vi "SubVI_ALD-Process-Step_Pulse_V16.vi"(0 "error in (no error)":errorcluster, 1 "Mod8 DAQ Name":tag, 2 "Mod7 DAQ Name":tag, 3 "Precursor Dose Array":T2={"Mod7"=[FALSE, FALSE, FALSE, FALSE, FALSE, FALSE, FALSE, FALSE], "Mod8"=[FALSE, FALSE, FALSE, FALSE, FALSE, FALSE, FALSE, FALSE]}, 5 "Precursor-i":i32, 7 "Precursor-i name":string, 9 "Dose Time (sec)":dbl, 12 "ProcessStep Input Cluster":T1, 14 "Recipe Step \nNumber":i32) -> (4 "error out":errorcluster, 8 "Dose Start Timestamp":timestamp, 15 "Execution Aborted \nDuring This Recipe Step?":bool)   [LabVIEW 2026]
uses:
  CTRL_DO Boolean Array Cluster_V16.ctl
panel:
  out "Dose Start Time":dbl
  # "NEED TO UPDATE SUBVI DESCRIPTION"
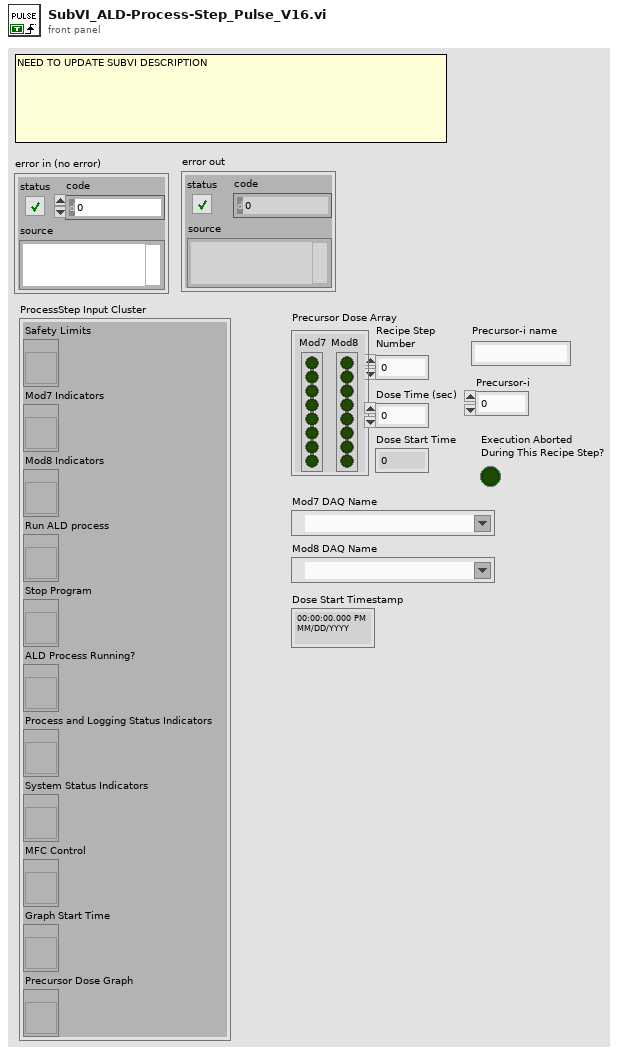
[diagram p1: front panel]
types:
  T1 = cluster{"Safety Limits":refnum<vi>, "Mod7 Indicators ":refnum<vi>, "Mod8 Indicators":refnum<vi>, "Run ALD process":refnum<vi>, "Stop Program":refnum<vi>, "ALD Process Running?":refnum<vi>, "Process and Logging Status Indicators":refnum<vi>, "System Status Indicators":refnum<vi>, "MFC Control":refnum<vi>, "Graph Start Time":refnum<vi>, "Precursor Dose Graph":refnum<vi>}
  T2 = typedef "CTRL_DO Boolean Array Cluster_V16.ctl" = cluster{"Mod7":bool[], "Mod8":bool[]}
  T3 = typedef "CTRL_ProcessLoggingStatusIndicator_V14.ctl" = cluster{"ALD Process Status:":string, "Logging Data to:":path, "Process Start Time:":string, "Process End Time:":string, "Steps Completed:":string}
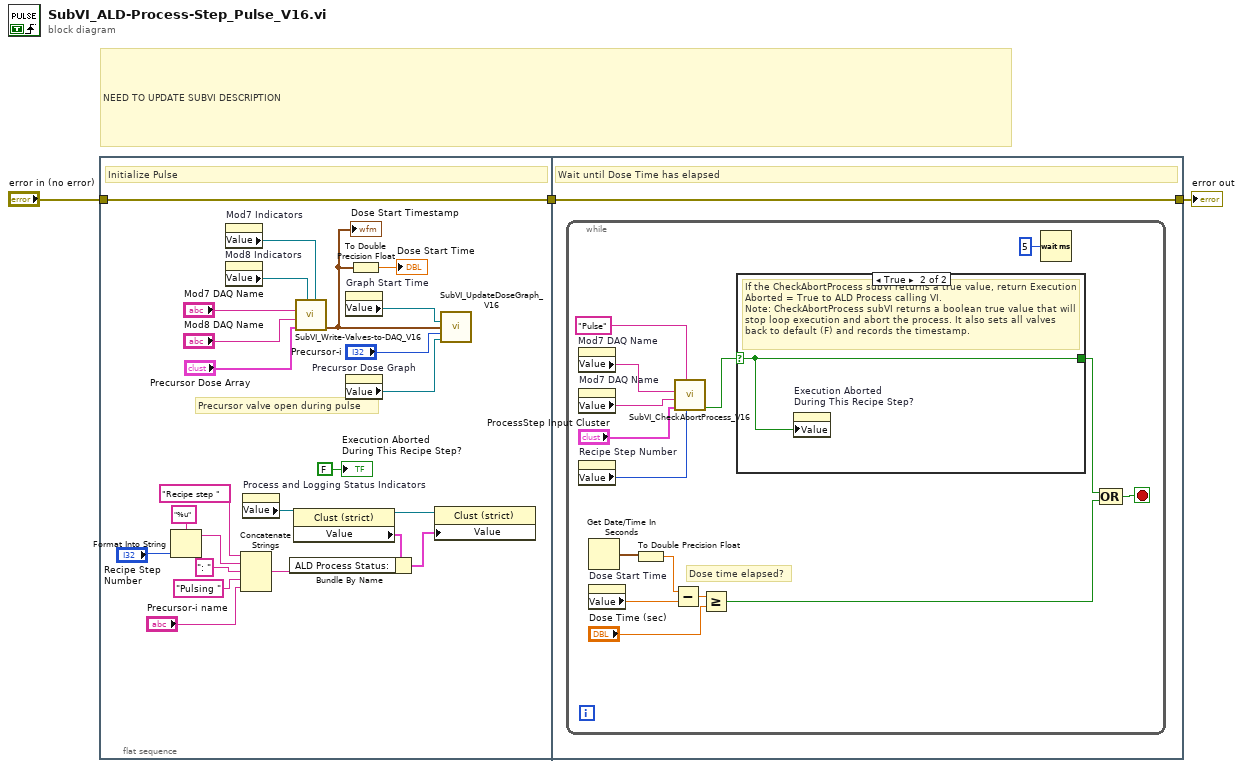
[diagram p0: block diagram]
diagram:
  # "NEED TO UPDATE SUBVI DESCRIPTION"
  n1 = flat-sequence {
    tunnel: "error in (no error)" -> [w26]
    tunnel: [w26] -> w1
    tunnel: [w28] -> w2
    tunnel: w1 -> [w28]
    frame #0 {
      # "Precursor valve open during pulse"
      # "Initialize Pulse"
      n2 = Format Into String(format string="%u", "Recipe Step \nNumber") -> (resulting string=w21:string)  [unwired: 2 in, 1 out]
      n3 = property on="Mod7 Indicators" class="LVObjRef (strict)"() -> ("Value"=w10:refnum<vi>)  [unwired: 2 in, 2 out]
      n4 = property on="Mod8 Indicators" class="LVObjRef (strict)"() -> ("Value"=w11:refnum<vi>)  [unwired: 2 in, 2 out]
      n5 = Concatenate Strings("Recipe step ", w21, ": " ("string"), "Pulsing " ("Value"), "Precursor-i name") -> (w24:string)
      n6 = property on="Process and Logging Status Indicators" class="LVObjRef (strict)"() -> ("Value"=w15:refnum<vi>)  [unwired: 2 in, 2 out]
      n7 = property class="Clust (strict)"(reference=w15) -> (reference out=w16:refnum<vi>, "Value"=w17:T3)  [unwired: 1 in, 1 out]
      n8 = Bundle By Name(cluster=w17, "ALD Process Status:"=w24) -> (w18:T3)
      n9 = call "SubVI_Write-Valves-to-DAQ_V16.vi"("Mod7 Indicators Ref"=w10, "Mod8 Indicators Ref"=w11, "DO Boolean Array Cluster"="Precursor Dose Array", "Mod8 Port Name"="Mod8 DAQ Name", "Mod7 Port Name"="Mod7 DAQ Name") -> ("current time"=w8:timestamp)  [unwired: 3 in, 3 out]
      "Dose Start Timestamp" <- w8
      n10 = property on="Graph Start Time" class="LVObjRef (strict)"() -> ("Value"=w7:refnum<vi>)  [unwired: 2 in, 2 out]
      n11 = property on="Precursor Dose Graph" class="LVObjRef (strict)"() -> ("Value"=w13:refnum<vi>)  [unwired: 2 in, 2 out]
      n12 = To Double Precision Float(number=w8) -> (double precision float=→"Dose Start Time":dbl)
      n13 = property class="Clust (strict)"(reference=w16, "Value"=w18) -> ()  [unwired: 1 in, 2 out]
      n14 = call "SubVI_UpdateDoseGraph_V16.vi"("Graph Start Time"=w7, "New Timestamp"=w8, "Precursor Valve Open"="Precursor-i", "Precursor Dose Graph"=w13) -> ()  [unwired: 11 in, 1 out]
      "Execution Aborted \nDuring This Recipe Step?" <- FALSE ("Execution Aborted?")
    }
    frame #1 {
      # "Wait until Dose Time has elapsed"
      n15 = while {
        stop <- w42 stop-if-true
        # "Dose time elapsed?"
        n16 = property on="Mod7 DAQ Name" class="DAQmxName"() -> ("Value"=w34:string)  [unwired: 2 in, 2 out]
        n17 = property on="Mod7 DAQ Name" class="DAQmxName"() -> ("Value"=w33:string)  [unwired: 2 in, 2 out]
        n18 = property on="Recipe Step Number" class="DigNum (strict)"() -> ("Value"=w32:i32)  [unwired: 2 in, 2 out]
        n19 = Get Date/Time In Seconds() -> (seconds since 1Jan1904=w38:timestamp)
        n20 = property on="Dose Start Time" class="DigNum (strict)"() -> ("Value"=w36:dbl)  [unwired: 2 in, 2 out]
        n21 = To Double Precision Float(number=w38) -> (double precision float=w37:dbl)
        n22 = Subtract(x=w37, y=w36) -> (x-y=w35:dbl)
        n23 = call "SubVI_CheckAbortProcess_V16.vi"("Process Step"=w32, "Step Description"="Pulse", "ProcessStep Input Cluster"="ProcessStep Input Cluster", "Mod8 DAQ Name"=w33, "Mod7 DAQ Name"=w34) -> ("Abort Process Execution"=w40:bool)  [unwired: 5 in, 1 out]
        n24 = Greater Or Equal?(x=w35, y="Dose Time (sec)") -> (x >= y?=w29:bool)
        n25 = case shown="True" w40 {
          selector: w40 -> [w44 w45]
          tunnel: [w44 w45] -> w41
          frame False {
            # "If the CheckAbortProcess subVI returns a false value, wait until Dose Time has elapsed."
          }
          frame True {
            # "If the CheckAbortProcess subVI returns a true value, return Execution Aborted = True to ALD Process calling VI. \nNote: CheckAbortProcess subVI returns a boolean true value that will stop loop execution and abort the process. It also sets all valves back to default (F) and records the timestamp."
            n26 = property on="Execution Aborted \nDuring This Recipe Step?" class="Bool (strict)"("Value"=w45) -> ()  [unwired: 2 in, 2 out]
          }
        }
        n27 = Wait (ms)(milliseconds to wait=u32 5) -> ()  [unwired: 1 out]
        n28 = Compound Arithmetic op=OR(w41, w29) -> (w42:bool)
      }
    }
  }
  "error out" <- w2
